vi "settle-detect.vi"(6 "error-max":sgl format="%#_13g", 8 "settled-samples\nthreshold":i16, 11 "err(k)":sgl) -> (0 "has-settled":bool, 3 "number-settled-samples":i16)   [LabVIEW 2017]
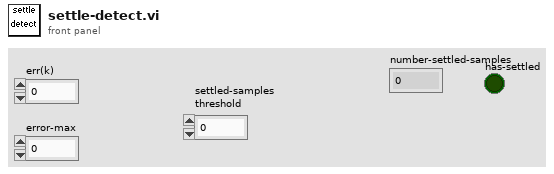
[diagram p1: front panel]
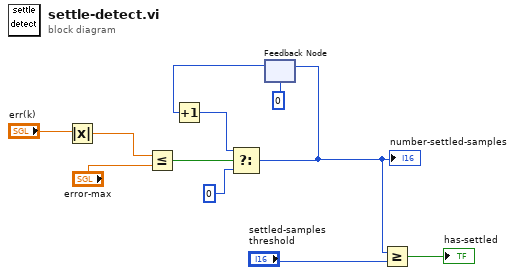
[diagram p0: block diagram]
diagram:
  n1 = Absolute Value(x="err(k)") -> (abs(x)=w2:sgl)
  n2 = Less Or Equal?(x=w2, y="error-max") -> (x <= y?=w7:bool)
  n3 = feedback #1(i16 0 ("f")) -> (w10:i16)
  n4 = Increment(x=w10) -> (x+1=w8:i16)
  n5 = Select(t=w8, s=w7, f=i16 0) -> (s? t:f=w5:i16)
  "number-settled-samples" <- w5
  n6 = feedback-in #1(w5) -> ()
  n7 = Greater Or Equal?(x=w5, y="settled-samples\nthreshold") -> (x >= y?=→"has-settled":bool)
